vi "Display_Image_From_File.vi"() -> ()   [LabVIEW 2017]
panel:
  out "error out":errorcluster
  out "Image":T1(plugin-control)
  out "Image File Selected":string
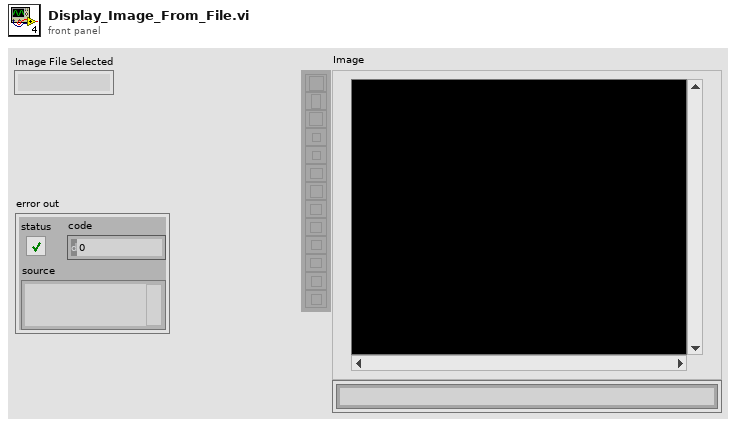
[diagram p1: front panel]
types:
  T1 = typedef "IMAQ Image.ctl" = refnum<image>
  T2 = typedef "Image Type" = u32
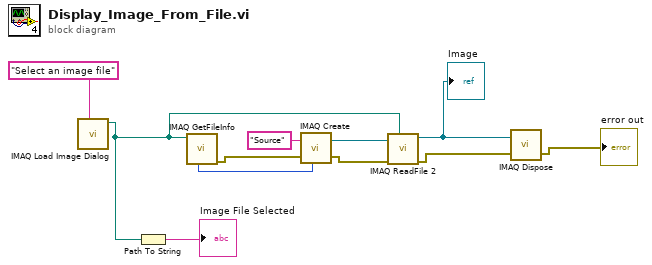
[diagram p0: block diagram]
diagram:
  n1 = call "IMAQ Load Image Dialog"("Prompt"="Select an image file") -> ("Path"=w4:path)  [unwired: 8 in, 2 out]
  n2 = Path To String(path=w4) -> (string=→"Image File Selected":string)
  n3 = call "IMAQ GetFileInfo"("File Path"=w4) -> ("error out"=w5:errorcluster, "Image Type"=w1:T2)  [unwired: 4 in, 5 out]
  n4 = call "IMAQ Create"("Image Name"="Source", "Image Type"=w1, "error in (no error)"=w5) -> ("New Image"=w3:T1, "error out"=w7:errorcluster)  [unwired: 2 in]
  n5 = call "IMAQ ReadFile 2"("File Path"=w4, "error in (no error)"=w7, "Image"=w3) -> ("error out"=w8:errorcluster, "Image Out"=w2:T1)  [unwired: 4 in, 3 out]
  "Image" <- w2
  n6 = call "IMAQ Dispose"("Image"=w2, "error in (no error)"=w8) -> ("error out"=→"error out":errorcluster)  [unwired: 4 in]
